vi "Function.vi"() -> ()   [LabVIEW 2019, in "LotCount.lvlib" / "LotCount.lvclass"]
uses:
  LotCount.lvclass
panel:
  out "text":string
  in  "Function":u8=2
  in  "Set_LotID":string
  in  "Set_Part":string
  in  "Set_Station":string
  out "Read_Station":string
  out "Read_LotID":string
  out "Read_Part":string
  out "Read_Number":i32=888
  out "Time":string="08/05/2020 15:06:23.664"
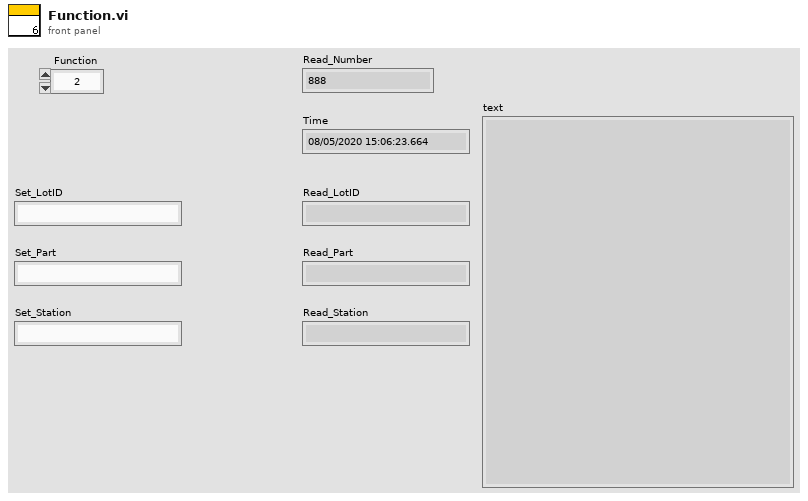
[diagram p1: front panel]
types:
  T1 = enum16{"open", "replace", "create", "open or create", "replace or create", "replace or create with confirmation"}
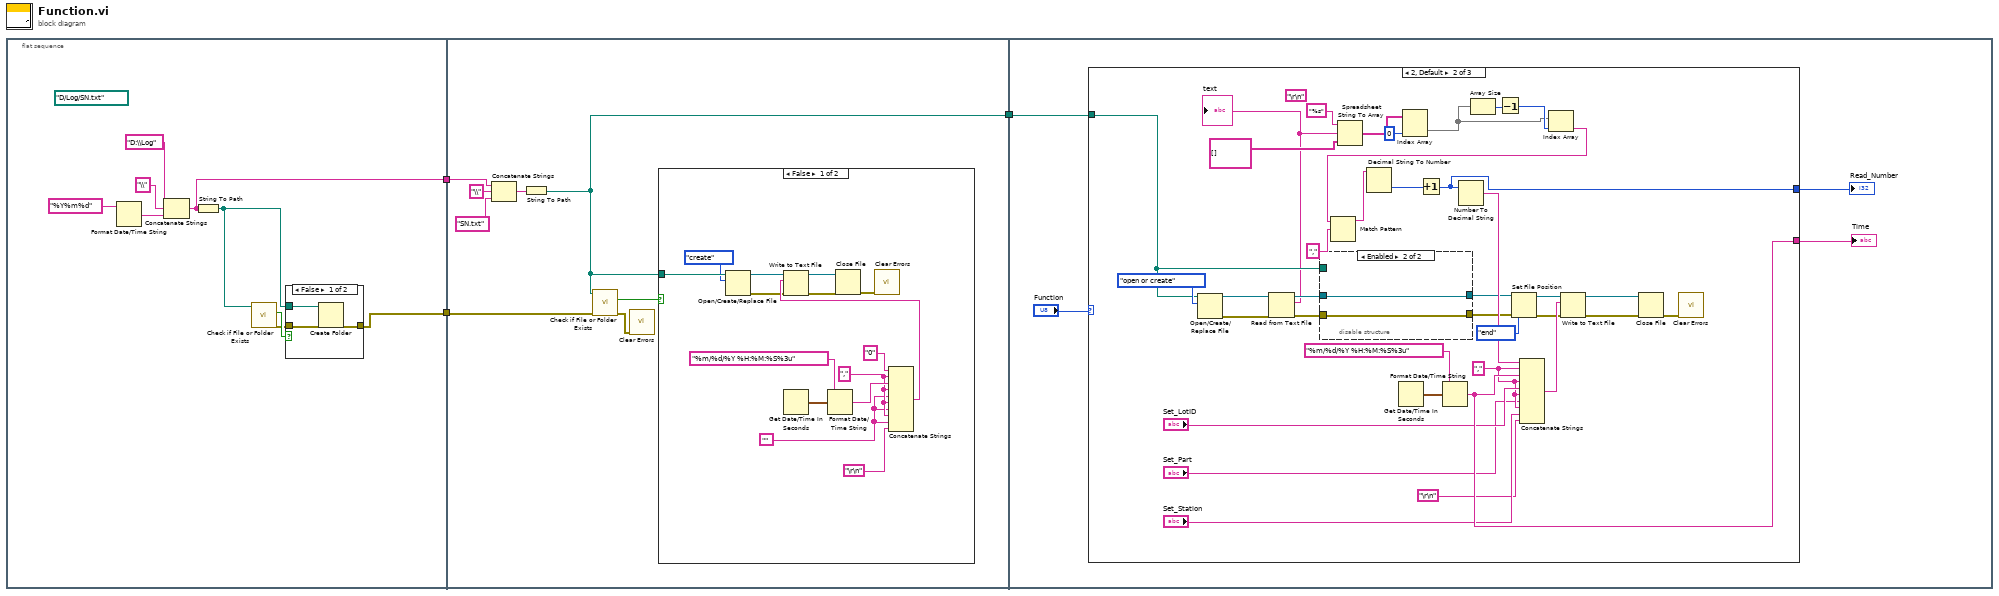
[diagram p0: block diagram]
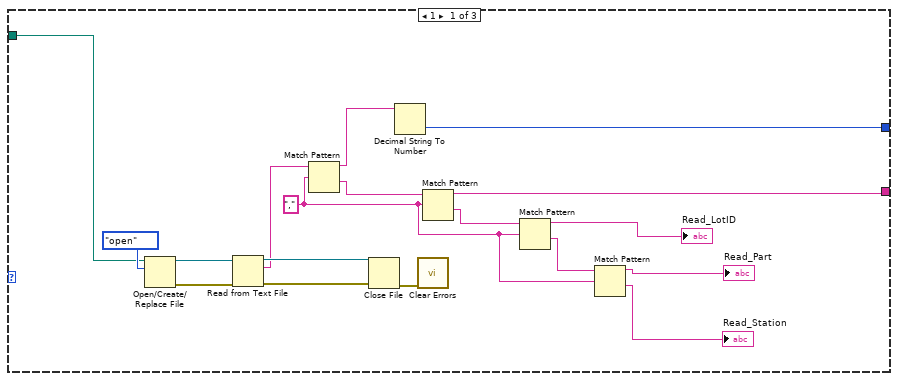
[diagram p4: hidden frame]
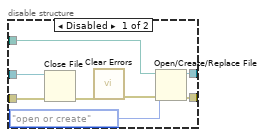
[diagram p5: hidden frame]
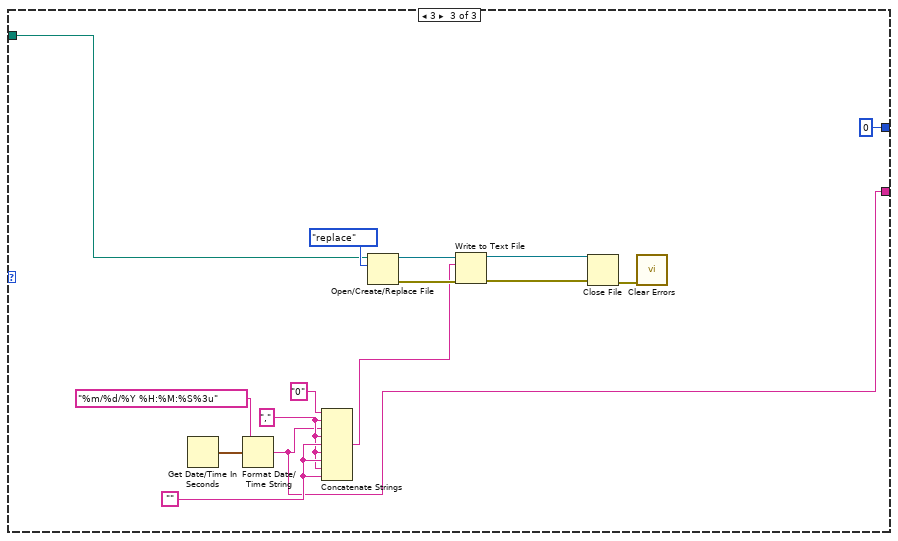
[diagram p6: hidden frame]
diagram:
  n1 = flat-sequence {
    tunnel: [w5] -> w2
    tunnel: [w4] -> w1
    tunnel: [w17] -> w3
    tunnel: w2 -> [w22]
    tunnel: w1 -> [w20]
    tunnel: w3 -> [w42]
    frame #0 {
      (unwired) path "D:/Log/SN.txt" ("path")
      n2 = Format Date/Time String(time format string (%c)="%Y%m%d") -> (date/time string=w10:string)  [unwired: 2 out]
      n3 = Concatenate Strings("D:\\Log" ("string"), "\\" ("string"), w10) -> (w4:string)
      n4 = String To Path(string=w4) -> (path=w6:path)
      n5 = call <vilib>:"Check if File or Folder Exists.vi"("path"=w6) -> ("error out"=w7:errorcluster, "file or folder exists?"=w8:bool)  [unwired: 1 in, 8 out]
      n6 = case shown="False" w8 {
        tunnel: w6 -> [w15 _]
        tunnel: w7 -> [w14 w16]
        tunnel: [w13 w16] -> w5
        frame False {
          n7 = Create Folder(path (use dialog)=w15, error in=w14) -> (error out=w13:errorcluster)  [unwired: 3 out]
        }
        frame True {
        }
      }
    }
    frame #1 {
      n8 = Concatenate Strings(w20, "\\" ("string"), "SN.txt" ("string")) -> (w18:string)
      n9 = String To Path(string=w18) -> (path=w17:path)
      n10 = call <vilib>:"Check if File or Folder Exists.vi"("error in (no error)"=w22, "path"=w17) -> ("error out"=w23:errorcluster, "file or folder exists?"=w24:bool)  [unwired: 7 in, 1 out]
      n11 = call <vilib>:"Clear Errors.vi"("error in (no error)"=w23) -> ()  [unwired: 5 in, 2 out]
      n12 = case shown="False" w24 {
        tunnel: w17 -> [w39 _]
        frame False {
          w26 = ""
          w27 = "," ("string")
          n13 = Open/Create/Replace File(file path (use dialog)=w39, operation (0:open)=T1."create") -> (refnum out=w32:refnum<file>, error out=w31:errorcluster)  [unwired: 4 in, 1 out]
          n14 = Get Date/Time In Seconds() -> (seconds since 1Jan1904=w36:timestamp)
          n15 = Format Date/Time String(time format string (%c)="%m/%d/%Y %H:%M:%S%3u", seconds (now)=w36) -> (date/time string=w34:string)  [unwired: 1 in]
          n16 = Concatenate Strings("0", w27, w34, w27, w26, w27, w26, w27, w26, "\r\n") -> (w33:string)
          n17 = Write to Text File(file (use dialog)=w32, text=w33, error in=w31) -> (refnum out=w29:refnum<file>, error out=w30:errorcluster)  [unwired: 1 in, 1 out]
          n18 = Close File(refnum=w29, error in=w30) -> (error out=w28:errorcluster)  [unwired: 1 out]
          n19 = call <vilib>:"Clear Errors.vi"("error in (no error)"=w28) -> ()  [unwired: 5 in, 2 out]
        }
        frame True {
        }
      }
    }
    frame #2 {
      n20 = case shown="2, Default" "Function" {
        tunnel: w42 -> [w54 w81 w118]
        tunnel: [w52 w83 0] -> w41
        tunnel: [w50 w84 w109] -> w40
        frame 1 {
          w47 = "," ("regular expression")
          n21 = Open/Create/Replace File(file path (use dialog)=w54, operation (0:open)=T1."open") -> (refnum out=w58:refnum<file>, error out=w60:errorcluster)  [unwired: 4 in, 1 out]
          n22 = Read from Text File(file (use dialog)=w58, error in=w60) -> (refnum out=w57:refnum<file>, text=w56:string, error out=w59:errorcluster)  [unwired: 2 in, 1 out]
          n23 = Match Pattern(string=w56, regular expression=w47) -> (before substring=w55:string, after substring=w51:string)  [unwired: 1 in, 2 out]
          n24 = Close File(refnum=w57, error in=w59) -> (error out=w53:errorcluster)  [unwired: 1 out]
          n25 = Decimal String To Number(string=w55) -> (number=w52:i32)  [unwired: 2 in, 1 out]
          n26 = call <vilib>:"Clear Errors.vi"("error in (no error)"=w53) -> ()  [unwired: 5 in, 2 out]
          n27 = Match Pattern(string=w51, regular expression=w47) -> (before substring=w50:string, after substring=w49:string)  [unwired: 1 in, 2 out]
          n28 = Match Pattern(string=w49, regular expression=w47) -> (before substring=→"Read_LotID":string, after substring=w46:string)  [unwired: 1 in, 2 out]
          n29 = Match Pattern(string=w46, regular expression=w47) -> (before substring=→"Read_Part":string, after substring=→"Read_Station":string)  [unwired: 1 in, 2 out]
        }
        frame 2, Default {
          (unwired) "\r\n"
          w79 = "," ("string")
          n30 = Open/Create/Replace File(file path (use dialog)=w81, operation (0:open)=T1."open or create") -> (refnum out=w96:refnum<file>, error out=w97:errorcluster)  [unwired: 4 in, 1 out]
          n31 = Read from Text File(file (use dialog)=w96, error in=w97) -> (refnum out=w82:refnum<file>, text=w69:string, error out=w89:errorcluster)  [unwired: 2 in, 1 out]
          "text" <- w69
          n32 = disable-structure shown="Enabled" {
            disable-tunnel: w89 -> [w106 w107]
            disable-tunnel: w82 -> [w105 w108]
            disable-tunnel: w81 -> [w104 _]
            disable-tunnel: [w100 w108] -> w75
            disable-tunnel: [w99 w107] -> w73
            frame Disabled {
              n33 = Close File(refnum=w105, error in=w106) -> (error out=w103:errorcluster)  [unwired: 1 out]
              n34 = call <vilib>:"Clear Errors.vi"("error in (no error)"=w103) -> ("error out"=w102:errorcluster)  [unwired: 5 in, 1 out]
              n35 = Open/Create/Replace File(file path (use dialog)=w104, error in=w102, operation (0:open)=T1."open or create") -> (refnum out=w100:refnum<file>, error out=w99:errorcluster)  [unwired: 3 in, 1 out]
            }
            frame Enabled {
            }
          }
          n36 = Spreadsheet String To Array(format string="%s", spreadsheet string=w69, array type (2D Dbl)=string[][] []) -> (array=w65:string[][])  [unwired: 1 in]
          n37 = Get Date/Time In Seconds() -> (seconds since 1Jan1904=w91:timestamp)
          n38 = Index Array(array=w65, index (col)=0 ("disabled index (col)")) -> (element=w63:string[])  [unwired: 1 in]
          n39 = Format Date/Time String(time format string (%c)="%m/%d/%Y %H:%M:%S%3u", seconds (now)=w91) -> (date/time string=w84:string)  [unwired: 1 in]
          n40 = Array Size(array=w63) -> (size(s)=w67:i32)
          n41 = Decrement(x=w67) -> (x-1=w66:i32)
          n42 = Set File Position(refnum=w75, from (0:start)=enum16{"start", "end", "current"}."end", error in=w73) -> (refnum out=w74:refnum<file>, error out=w72:errorcluster)  [unwired: 1 out]
          n43 = Index Array(array=w63, index=w66) -> (element=w62:string)
          n44 = Match Pattern(string=w62, regular expression=",") -> (before substring=w94:string)  [unwired: 1 in, 3 out]
          n45 = Decimal String To Number(string=w94) -> (number=w92:i32)  [unwired: 2 in, 1 out]
          n46 = Increment(x=w92) -> (x+1=w83:i32)
          n47 = Number To Decimal String(number=w83) -> (decimal integer string=w86:string)  [unwired: 1 in]
          n48 = Concatenate Strings(w86, w79, w84, w79, "Set_LotID", w79, "Set_Part", w79, "Set_Station", "\r\n") -> (w85:string)
          n49 = Write to Text File(file (use dialog)=w74, text=w85, error in=w72) -> (refnum out=w87:refnum<file>, error out=w88:errorcluster)  [unwired: 1 in, 1 out]
          n50 = Close File(refnum=w87, error in=w88) -> (error out=w93:errorcluster)  [unwired: 1 out]
          n51 = call <vilib>:"Clear Errors.vi"("error in (no error)"=w93) -> ()  [unwired: 5 in, 2 out]
        }
        frame 3 {
          w115 = ""
          w114 = "," ("string")
          n52 = Get Date/Time In Seconds() -> (seconds since 1Jan1904=w112:timestamp)
          n53 = Format Date/Time String(time format string (%c)="%m/%d/%Y %H:%M:%S%3u", seconds (now)=w112) -> (date/time string=w109:string)  [unwired: 1 in]
          n54 = Concatenate Strings("0", w114, w109, w114, w115, w114, w115, w114, w115) -> (w110:string)
          n55 = Open/Create/Replace File(file path (use dialog)=w118, operation (0:open)=T1."replace") -> (refnum out=w120:refnum<file>, error out=w122:errorcluster)  [unwired: 4 in, 1 out]
          n56 = Write to Text File(file (use dialog)=w120, text=w110, error in=w122) -> (refnum out=w119:refnum<file>, error out=w121:errorcluster)  [unwired: 1 in, 1 out]
          n57 = Close File(refnum=w119, error in=w121) -> (error out=w117:errorcluster)  [unwired: 1 out]
          n58 = call <vilib>:"Clear Errors.vi"("error in (no error)"=w117) -> ()  [unwired: 5 in, 2 out]
        }
      }
      "Read_Number" <- w41
      "Time" <- w40
    }
  }
